vi "Linear_Chart_Formula.vi"(3 "Max Voltage":dbl, 7 "Start":refnum<vi>, 8 "error in (no error)":errorcluster, 10 "Start":bool, 11 "Min Voltage":dbl) -> (0 "error out":errorcluster)   [LabVIEW 2020]
uses:
  Global 1.vi
panel:
  out "Remove initial zero":dbl[](array[numeric])
  out "size(s)":i32
  out "BeforeChange":dbl[](array[numeric])
  out "Output Array":dbl[](array[numeric])
  out "XY Graph":cluster{"X":dbl, "Y":dbl}[](graph)
  in  "Number of Steps \n(Liner Voltage ONLY)":dbl
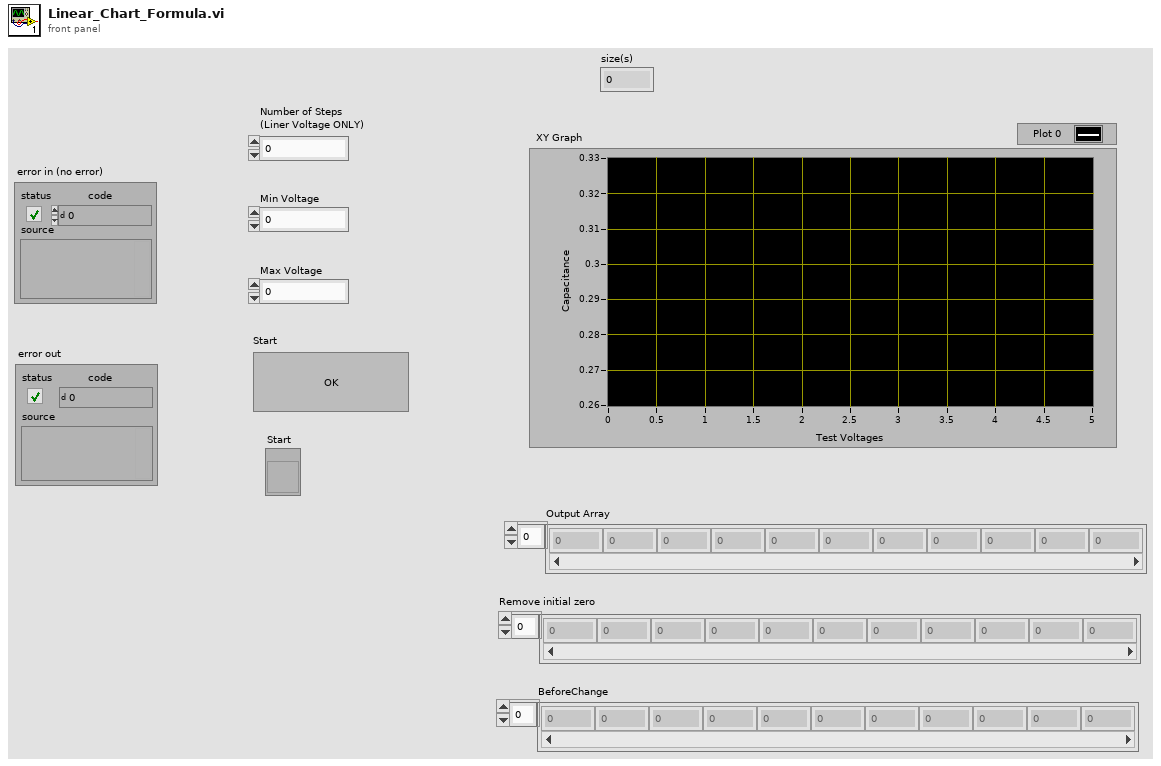
[diagram p1: front panel]
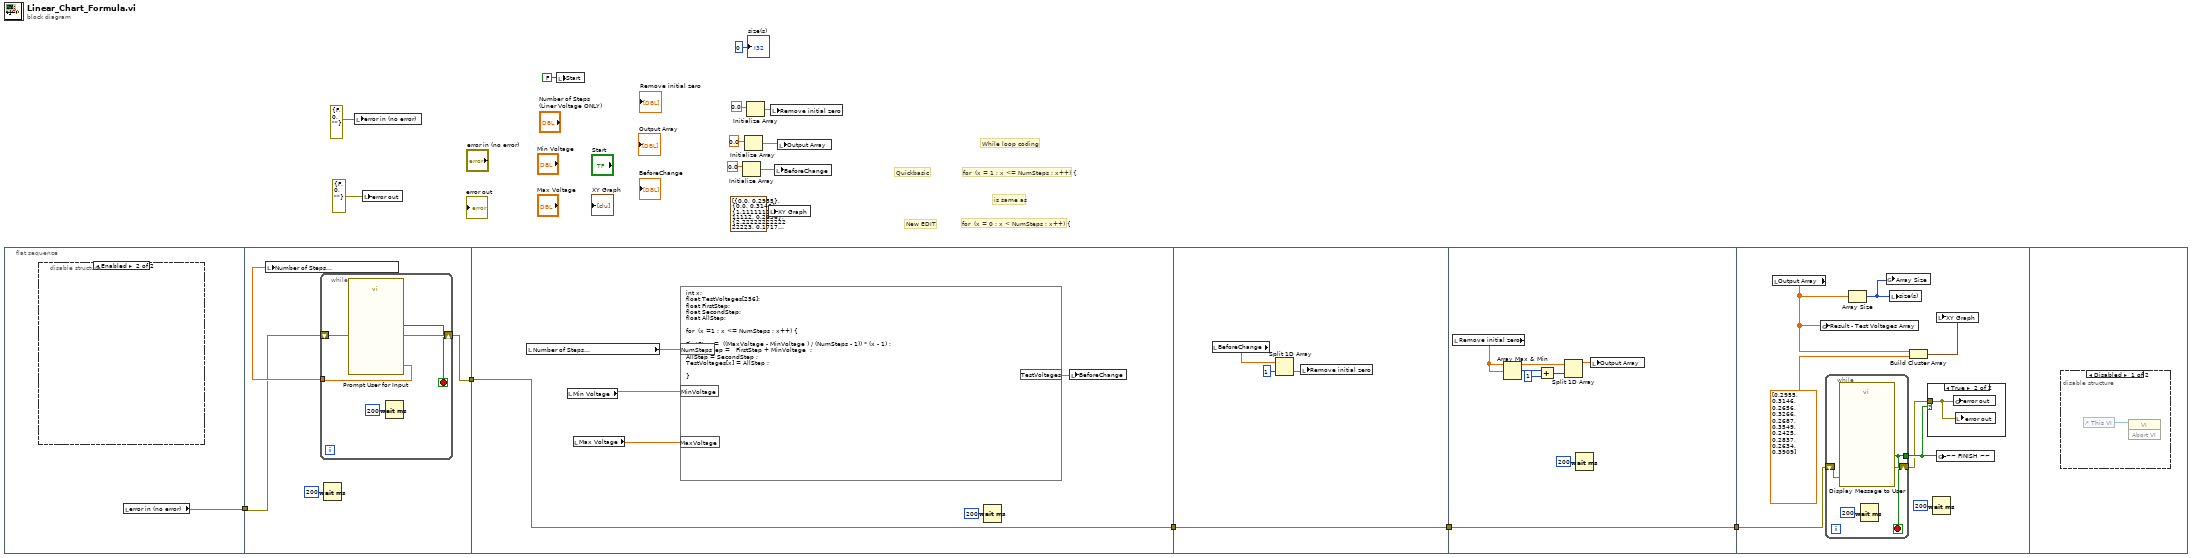
[diagram p0: block diagram]
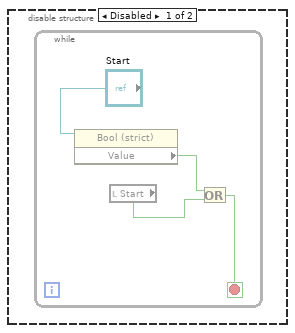
[diagram p2: hidden frame]
diagram:
  # "New EDIT"
  # "Quickbasic"
  # "for  (x = 0 ; x < NumSteps ; x++) {"
  # "is same as"
  # "for  (x = 1 ; x <= NumSteps ; x++) {"
  # "While loop coding"
  n1 = flat-sequence {
    tunnel: [w17] -> w10
    tunnel: w10 -> [w23]
    tunnel: [w22] -> w6
    tunnel: [w31] -> w2
    tunnel: w6 -> [w31]
    tunnel: w2 -> [w40]
    tunnel: [w40] -> w1
    tunnel: [w41] -> w7
    tunnel: w1 -> [w41]
    tunnel: w7 -> [w53]
    frame #0 {
      n2 = disable-structure shown="Enabled" {
        frame Disabled {
          n3 = while {
            stop <- w19 stop-if-true
            n4 = property class="Bool (strict)"(reference="Start") -> ("Value"=w21:bool)  [unwired: 1 in, 2 out]
            n5 = local read "Start"() -> (w20:bool)
            n6 = Or(x=w21, y=w20) -> (x .or. y?=w19:bool)
          }
        }
        frame Enabled {
        }
      }
      n7 = local read "error in (no error)"() -> (w17:errorcluster)
    }
    frame #1 {
      n8 = while {
        tunnel: [w26] -> w24
        shift-right: [w29] -> w22
        shift-left: w23 -> [w30]
        stop <- w28 stop-if-true
        n9 = call "Prompt User for Input"("error in (no error)"=w30) -> ("NUMSTEPS"=w26:dbl, "OK"=w28:bool, "error out"=w29:errorcluster)  [unwired: 16 in]
        n10 = Wait (ms)(milliseconds to wait=u32 200) -> ()  [unwired: 1 out]
      }
      n11 = local write "Number of Steps \n(Liner Voltage ONLY)"(w24) -> ()
      n12 = Wait (ms)(milliseconds to wait=u32 200) -> ()  [unwired: 1 out]
    }
    frame #2 {
      n13 = local read "Number of Steps \n(Liner Voltage ONLY)"() -> (w35:dbl)
      n14 = local read "Min Voltage"() -> (w34:dbl)
      n15 = local read "Max Voltage"() -> (w33:dbl)
      n16 = formula code="int x;\nfloat TestVoltages[256];\nfloat FirstStep;\nfloat SecondStep;\nfloat AllStep;\n\nfor  (x =1 ; x <= NumSteps ; x++) {\n\nFirstStep =  ((MaxVoltage - MinVoltage ) / (NumSteps - 1)) * (x - 1) ;\nSecondStep =   FirstStep + MinVoltage  ;\nAllStep = SecondStep ;\nTestVoltages[x] = AllStep ;\n\n}"("NumSteps"=w35, "MinVoltage"=w34, "MaxVoltage"=w33) -> ("TestVoltages"=w32:dbl[])
      n17 = Wait (ms)(milliseconds to wait=u32 200) -> ()  [unwired: 1 out]
      n18 = local write "BeforeChange"(w32) -> ()
    }
    frame #3 {
      n19 = local read "BeforeChange"() -> (w39:dbl[])
      n20 = Split 1D Array(array=w39, index=1) -> (second subarray=w38:dbl[])  [unwired: 1 out]
      n21 = local write "Remove initial zero"(w38) -> ()
    }
    frame #4 {
      n22 = local read "Remove initial zero"() -> (w44:dbl[])
      n23 = Array Max & Min(array=w44) -> (max index (indices)=w47:i32)  [unwired: 3 out]
      n24 = Add(x=w47, y=1) -> (x+y=w45:i32)
      n25 = Split 1D Array(array=w44, index=w45) -> (first subarray=w43:dbl[])  [unwired: 1 out]
      n26 = Wait (ms)(milliseconds to wait=u32 200) -> ()  [unwired: 1 out]
      n27 = local write "Output Array"(w43) -> ()
    }
    frame #5 {
      n28 = local read "Output Array"() -> (w52:dbl[])
      n29 = global write "Global 1.vi" "Result - Test Voltages Array"(w52) -> ()
      n30 = while {
        tunnel: [w56] -> w50
        shift-right: [w58] -> w49
        shift-left: w53 -> [w59]
        stop <- w56 stop-if-true
        n31 = call "Display Message to User"("error in (no error)"=w59) -> ("error out"=w58:errorcluster, "OK"=w56:bool)  [unwired: 9 in]
        n32 = Wait (ms)(milliseconds to wait=u32 200) -> ()  [unwired: 1 out]
      }
      n33 = Array Size(array=w52) -> (size(s)=w51:i32)
      n34 = global write "Global 1.vi" "Array Size"(w51) -> ()
      n35 = local write "size(s)"(w51) -> ()
      n36 = Build Cluster Array ("Index & Bundle Cluster Array")(w52, dbl[] [0.2955, 0.3146, 0.2656, 0.3266, 0.2687, 0.3549, 0.2425, 0.2837, 0.2634, 0.3909]) -> (w54:cluster{"Numeric":dbl, dbl}[])
      n37 = case shown="True" w50 {
        tunnel: w49 -> [_ w60]
        frame False {
        }
        frame True {
          n38 = global write "Global 1.vi" "error out"(w60) -> ()
          n39 = local write "error out"(w60) -> ()
        }
      }
      n40 = Wait (ms)(milliseconds to wait=u32 200) -> ()  [unwired: 1 out]
      n41 = local write "XY Graph"(w54) -> ()
      n42 = global write "Global 1.vi" "~~ FINISH ~~"(w50) -> ()
    }
    frame #6 {
      n43 = disable-structure shown="Disabled" {
        frame Disabled {
          n44 = control-ref of="This VI"() -> (w61:refnum<vi>)
          n45 = invoke class="VI" method="Abort VI"(reference=w61) -> ()  [unwired: 2 in, 3 out]
        }
        frame Enabled {
        }
      }
    }
  }
  n46 = local write "error in (no error)"(errorcluster {"status"=FALSE, "code"=0, "source"=""} ("error out")) -> ()
  n47 = local write "error out"(errorcluster {"status"=FALSE, "code"=0, "source"=""} ("error in (no error)")) -> ()
  n48 = local write "Start"(FALSE ("Start")) -> ()
  n49 = Initialize Array(0.0 ("element")) -> (w14:dbl[])  [unwired: 1 in]
  n50 = Initialize Array(0.0 ("element")) -> (w15:dbl[])  [unwired: 1 in]
  n51 = Initialize Array(0.0 ("element")) -> (w4:dbl[])  [unwired: 1 in]
  n52 = local write "XY Graph"(cluster{"X":dbl, "Y":dbl}[] [{"X"=0.0, "Y"=0.2955}, {"X"=0.0, "Y"=0.3146}, {"X"=1.1111111111111112, "Y"=0.2656}, {"X"=2.2222222222222223, "Y"=0.1717}, {"X"=3.3333333333333335, "Y"=0.2687}, {"X"=4.444444444444445, "Y"=0.3549}, {"X"=5.555555555555555, "Y"=0.2425}, {"X"=6.666666666666667, "Y"=0.2837}, {"X"=7.777777777777779, "Y"=0.2634}, {"X"=8.88888888888889, "Y"=0.3909}] ("XY Graph")) -> ()
  n53 = local write "Remove initial zero"(w4) -> ()
  n54 = local write "BeforeChange"(w14) -> ()
  n55 = local write "Output Array"(w15) -> ()
  "size(s)" <- 0 ("size(s)")
